vi "pmu_Buffer Waveforms.vi"(0 "data in":T2, 1 "frequency configuration":T4={"channel index"=0, "nominal Fs/actual Fs"=1.0}, 2 "reset? (F)":bool, 5 "GPS information":T1[](array[typedef]), 7 "unlocked first index":i32, 9 "system info in":refnum<class "PMU System Info.lvclass">, 11 "error in (no error)":errorcluster) -> (3 "samples to read":u32, 4 "reporting raw data":T3, 6 "buffered zero-crossing frequency":T5, 8 "reporting GPS information":T1, 10 "system info out":refnum<class "PMU System Info.lvclass">, 15 "error out":errorcluster)   [LabVIEW 2013, in "NI_EP_PMU.lvlib"]
doc: "Determines whether a GPS signal is locked. Once a GPS signal is locked, this VI writes <b>waveforms in</b> to a circular buffer and calculates <b>elements to read</b> for the next cycle."
uses:
  <vilib>/addons/Electrical Power/PMU/NI_EP_PMU.lvlib
  <vilib>/addons/Electrical Power/PMU/Common/Classes/PMU System Info/PMU System Info.lvclass
  <vilib>/addons/Electrical Power/PMU/Common/Controls/pmu_Phasor Measurement Data.ctl
  <vilib>/addons/Electrical Power/PMU/Common/Controls/pmu_GPS Info.ctl
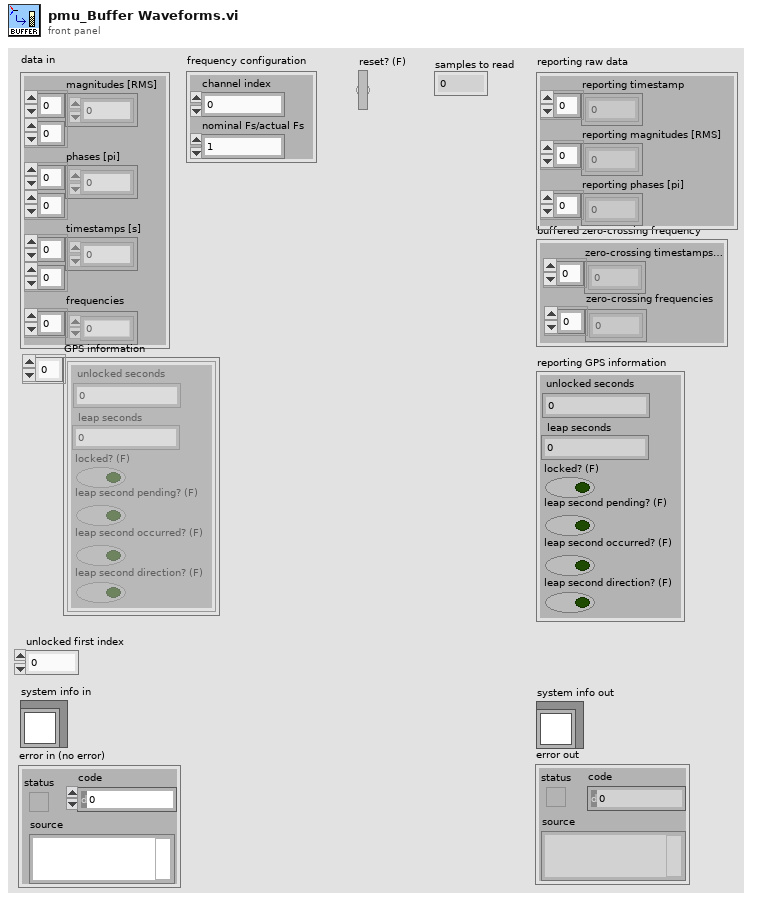
[diagram p1: front panel]
types:
  T1 = typedef "NI_EP_PMU.lvlib/pmu_GPS Info.ctl" = cluster{"unlocked seconds":u32, "leap seconds":i8, "locked? (F)":bool, "leap second pending? (F)":bool, "leap second occurred? (F)":bool, "leap second direction? (F)":bool}
  T2 = typedef "NI_EP_PMU.lvlib/pmu_Phasor Measurement Data.ctl" = cluster{"magnitudes [RMS]":dbl[][], "phases [pi]":dbl[][], "timestamps [s]":dbl[][], "frequencies":dbl[]}
  T3 = cluster{"reporting timestamp":dbl[], "reporting magnitudes [RMS]":dbl[], "reporting phases [pi]":dbl[]}
  T4 = cluster{"channel index":i32, "nominal Fs/actual Fs":dbl}
  T5 = cluster{"zero-crossing timestamps [s]":dbl[], "zero-crossing frequencies":dbl[]}
  T6 = typedef "NI_EP_PMU.lvlib/pmu_ROCOF Detector Settings.ctl" = cluster{"ROCOF window width":i32}
  T7 = typedef "NI_EP_PMU.lvlib/pmu_CFG Class.ctl" = cluster{"station name":string, "PMU ID":u16, "time base":u32, "nominal frequency":enum16{"50 Hz", "60 Hz"}, "reporting rate":i16, "phasor number":u16, "analog number":u16, "digital number":u16, "channel names":string[], "phasor units":u32[], "analog units":u32[], "digital units":u32[], "data format":u16, "number of PMUs":u16}
  T8 = cluster{"zero-crossing timestamps":dbl[], "zero-crossing frequencies":dbl[]}
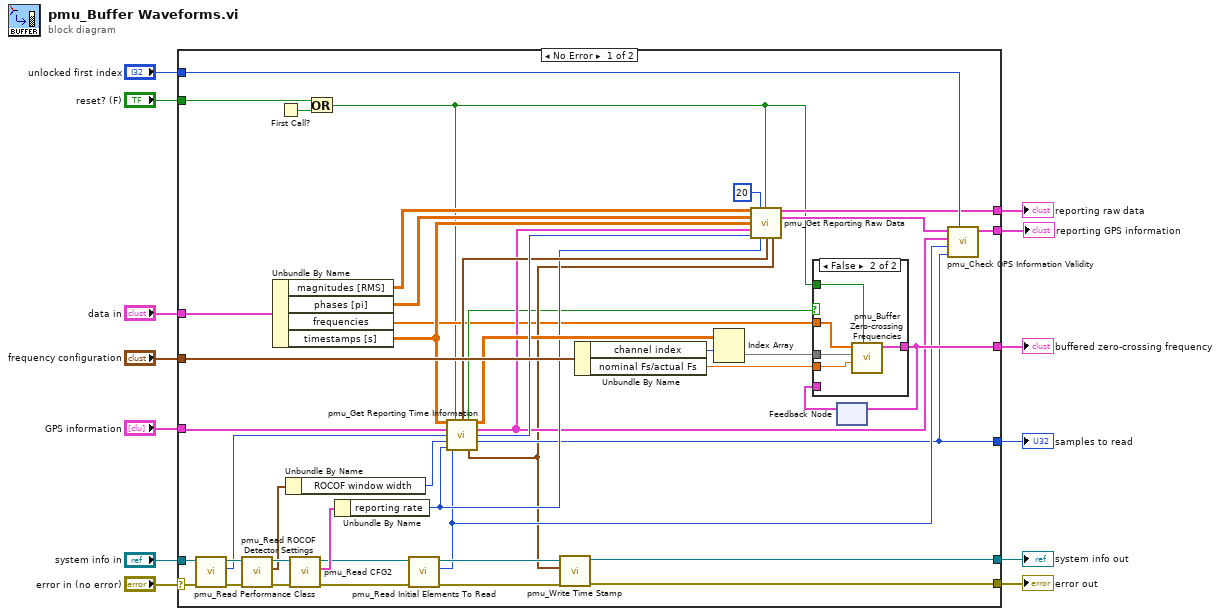
[diagram p0: block diagram]
diagram:
  n1 = case shown="No Error" "error in (no error)" {
    selector: "error in (no error)" -> [w16 w65]
    tunnel: "reset? (F)" -> [w41 _]
    tunnel: "data in" -> [w49 _]
    tunnel: "system info in" -> [w55 w66]
    tunnel: "frequency configuration" -> [w57 _]
    tunnel: [w50 _] -> w9
    tunnel: [w33 w65] -> w8
    tunnel: [w34 w66] -> w7
    tunnel: [w28 _] -> w6
    tunnel: [w24 _] -> w5
    tunnel: "GPS information" -> [w42 _]
    tunnel: [w30 _] -> w2
    tunnel: "unlocked first index" -> [w32 _]
    frame No Error {
      n2 = call <vilib>:"pmu_Read Performance Class.vi"("error in (no error)"=w16, "system info in"=w55) -> ("error out"=w15:errorcluster, "performance class"=w14:enum16{"M Class", "P Class"}, "system info out"=w17:refnum<class "PMU System Info.lvclass">)  [unwired: 7 in]
      n3 = call <vilib>:"pmu_Read ROCOF Detector Settings.vi"("error in (no error)"=w15, "system info in"=w17) -> ("error out"=w54:errorcluster, "ROCOF detector settings"=w52:T6, "system info out"=w53:refnum<class "PMU System Info.lvclass">)  [unwired: 7 in]
      n4 = Unbundle By Name(w49) -> ("magnitudes [RMS]"=w48:dbl[][], "phases [pi]"=w47:dbl[][], "frequencies"=w20:dbl[], "timestamps [s]"=w46:dbl[][])
      n5 = First Call?() -> (First Call?: T/F=w40:bool)
      n6 = Unbundle By Name(w52) -> ("ROCOF window width"=w27:i32)
      n7 = call <vilib>:"pmu_Read CFG2.vi"("error in (no error)"=w54, "system info in"=w53) -> ("error out"=w38:errorcluster, "CFG-2"=w58:T7, "system info out"=w39:refnum<class "PMU System Info.lvclass">)  [unwired: 7 in]
      n8 = Or(x=w41, y=w40) -> (x .or. y?=w19:bool)
      n9 = Unbundle By Name(w58) -> ("reporting rate"=w35:i16)
      n10 = call <vilib>:"pmu_Read Initial Elements To Read.vi"("error in (no error)"=w38, "system info in"=w39) -> ("error out"=w37:errorcluster, "initial elements to read"=w29:u32, "system info out"=w36:refnum<class "PMU System Info.lvclass">)  [unwired: 7 in]
      n11 = call <vilib>:"pmu_Get Reporting Time Information.vi"("timestamps in"=w46, "reset? (F)"=w19, "GPS information in"=w42, "performance class"=w14, "windows length"=w27, "reporting rate"=w35, "initial samples to read"=w29) -> ("min final timestamp"=w43:timestamp, "empty?"=w22:bool, "timestamps out"=w44:dbl[][], "GPS information out"=w31:T1[], "max t0 index"=w45:i32, "samples to read"=w28:u32, "current reporting time"=w26:timestamp)  [unwired: 2 in]
      n12 = call <vilib>:"pmu_Write Time Stamp.vi"("error in (no error)"=w37, "time stamp"=w26, "system info in"=w36) -> ("error out"=w33:errorcluster, "system info out"=w34:refnum<class "PMU System Info.lvclass">)  [unwired: 7 in]
      n13 = Unbundle By Name(w57) -> ("channel index"=w56:i32, "nominal Fs/actual Fs"=w18:dbl)
      n14 = Index Array(array=w44, index (row)=w56) -> (element=w51:dbl[])  [unwired: 1 in]
      n15 = call <vilib>:"pmu_Get Reporting Raw Data.vi"("magnitudes [RMS]"=w48, "buffer length"=20, "reset? (F)"=w19, "phases [pi]"=w47, "timestamps out"=w46, "buffered GPS information"=w31, "max t0 index"=w45, "reporting rate"=w35, "min final timestamp"=w43, "current reporting time"=w26) -> ("reporting raw data"=w24:T3, "reporting GPS information"=w23:T1)  [unwired: 4 in]
      n16 = feedback #1() -> (w25:T8)  [unwired: 1 in]
      n17 = case shown="False" w22 {
        tunnel: w51 -> [_ w64]
        tunnel: [w59 w63] -> w50
        tunnel: w20 -> [_ w62]
        tunnel: w19 -> [_ w61]
        tunnel: w25 -> [w59 _]
        tunnel: w18 -> [_ w60]
        frame True {
        }
        frame False {
          n18 = call <vilib>:"pmu_Buffer Zero-crossing Frequencies.vi"("Reset? (F)"=w61, "nominal Fs/actual Fs"=w60, "timestamps out"=w64, "frequencies"=w62) -> ("buffered zero-crossing frequency"=w63:T8)  [unwired: 7 in]
        }
      }
      n19 = feedback-in #1(w50) -> ()
      n20 = call <vilib>:"pmu_Check GPS Information Validity.vi"("unlocked first index"=w32, "samples to read"=w28, "initial samples to read"=w29, "GPS information"=w31, "reporting GPS information in"=w23) -> ("reporting GPS information out"=w30:T1)  [unwired: 6 in]
    }
    frame Error {
    }
  }
  "error out" <- w8
  "system info out" <- w7
  "buffered zero-crossing frequency" <- w9
  "samples to read" <- w6
  "reporting raw data" <- w5
  "reporting GPS information" <- w2
